vi "Draw Resize Box.vi"(0 "CtrlRef":refnum<vi>, 1 "Corners":refnum<vi>[](array[refnum]), 2 "ID":string, 3 "This VI":refnum<vi>, 5 "Origin":T3, 7 "Coords":T3, 9 "Size":T2, 13 "Active?":bool, 14 "Window Bounds":T1) -> ()   [LabVIEW 2011]
uses:
  <vilib>/Utility/miscctls.llb/LVPoint32TypeDef.ctl
  <vilib>/Utility/miscctls.llb/LVBoundsTypeDef.ctl
  <vilib>/Utility/miscctls.llb/LVRectTypeDef.ctl
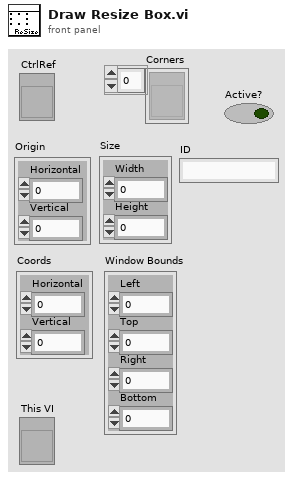
[diagram p1: front panel]
types:
  T1 = typedef "LVRectTypeDef.ctl" = cluster{"Left":i16, "Top":i16, "Right":i16, "Bottom":i16}
  T2 = typedef "LVBoundsTypeDef.ctl" = cluster{"Width":u32, "Height":u32}
  T3 = typedef "LVPoint32TypeDef.ctl" = cluster{"Horizontal":i32, "Vertical":i32}
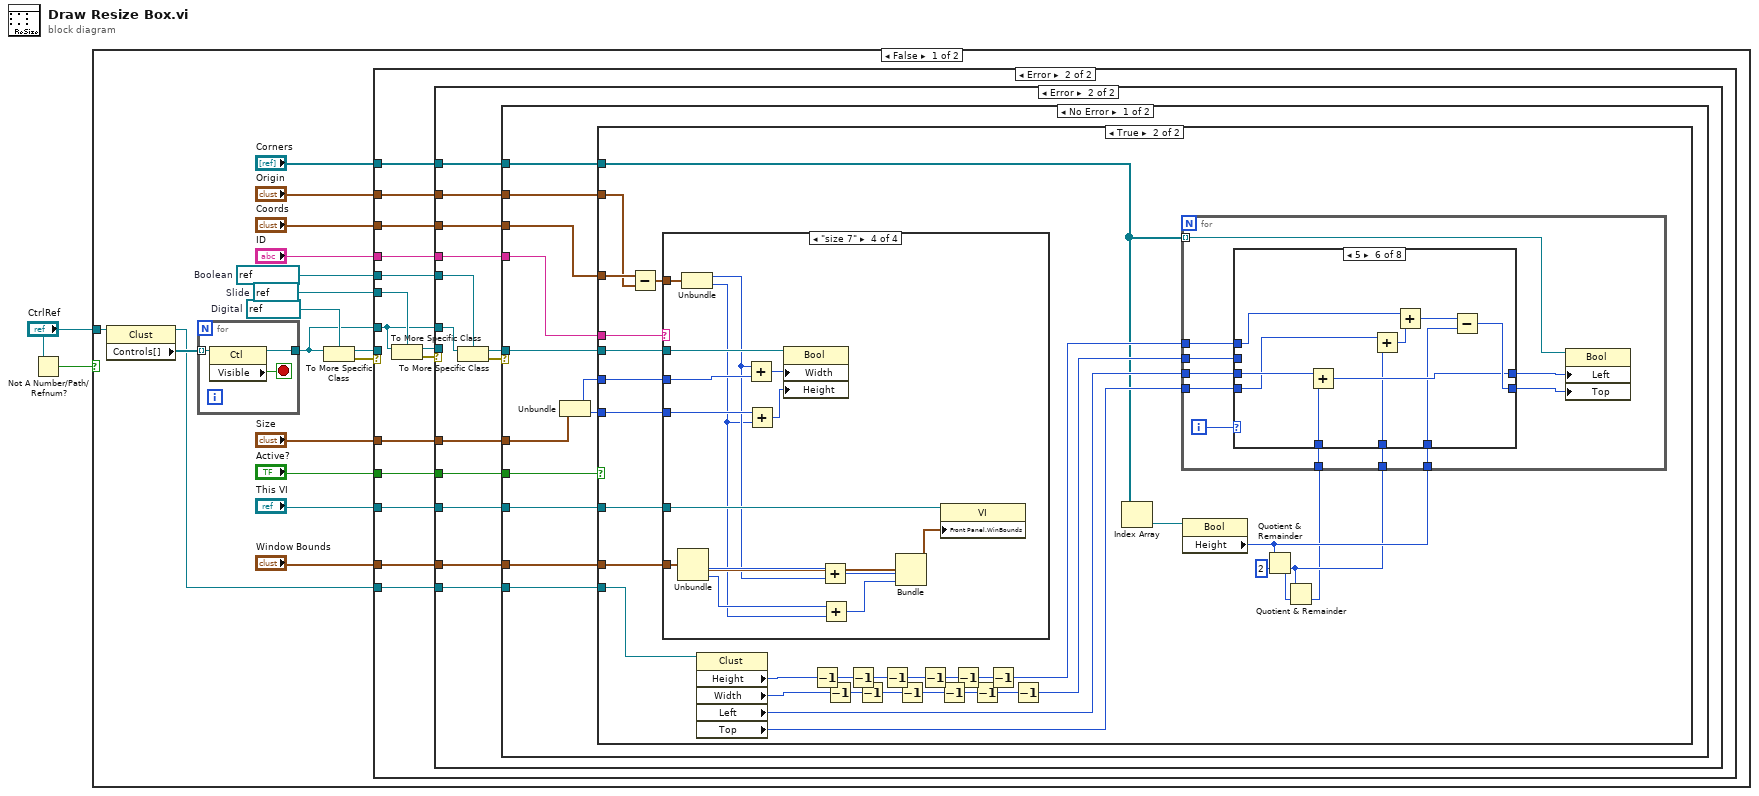
[diagram p0: block diagram]
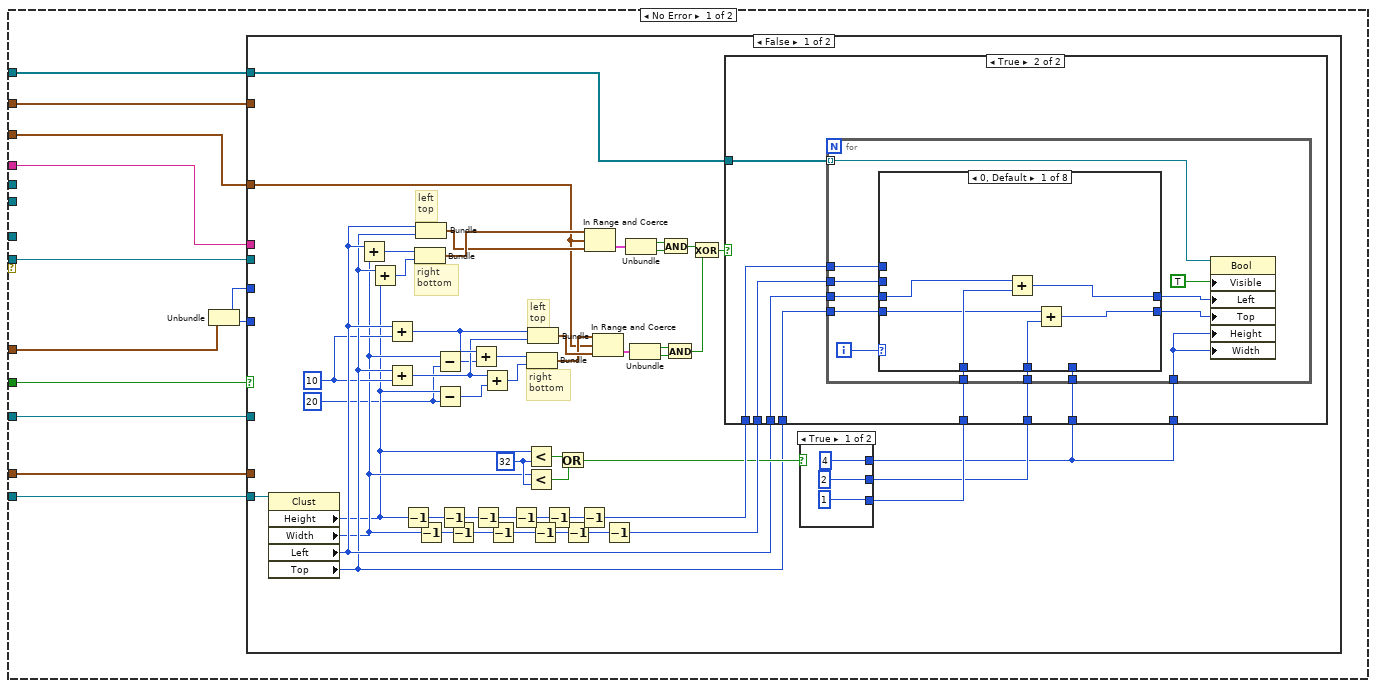
[diagram p2: hidden frame]
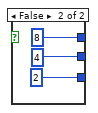
[diagram p3: hidden frame]
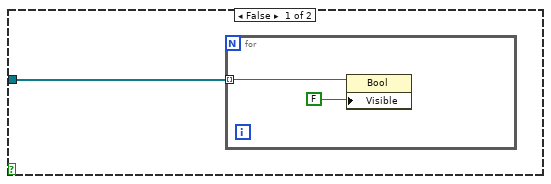
[diagram p4: hidden frame]
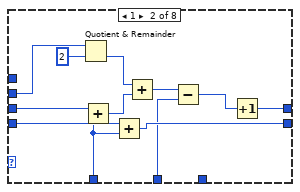
[diagram p5: hidden frame]
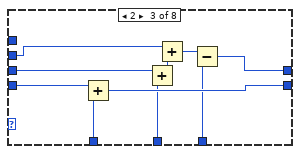
[diagram p6: hidden frame]
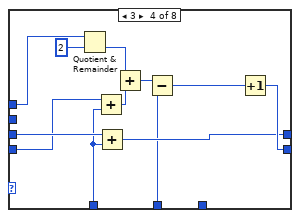
[diagram p7: hidden frame]
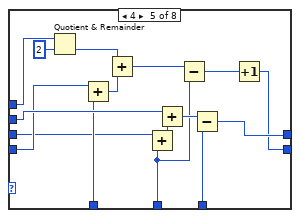
[diagram p8: hidden frame]
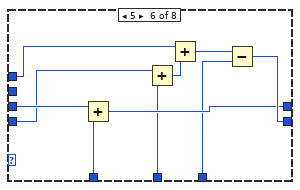
[diagram p9: hidden frame]
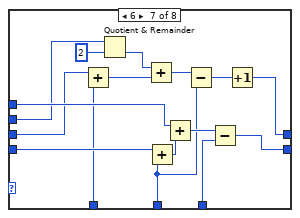
[diagram p10: hidden frame]
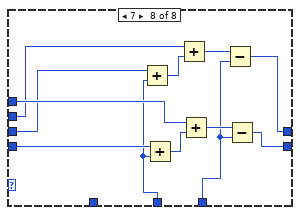
[diagram p11: hidden frame]
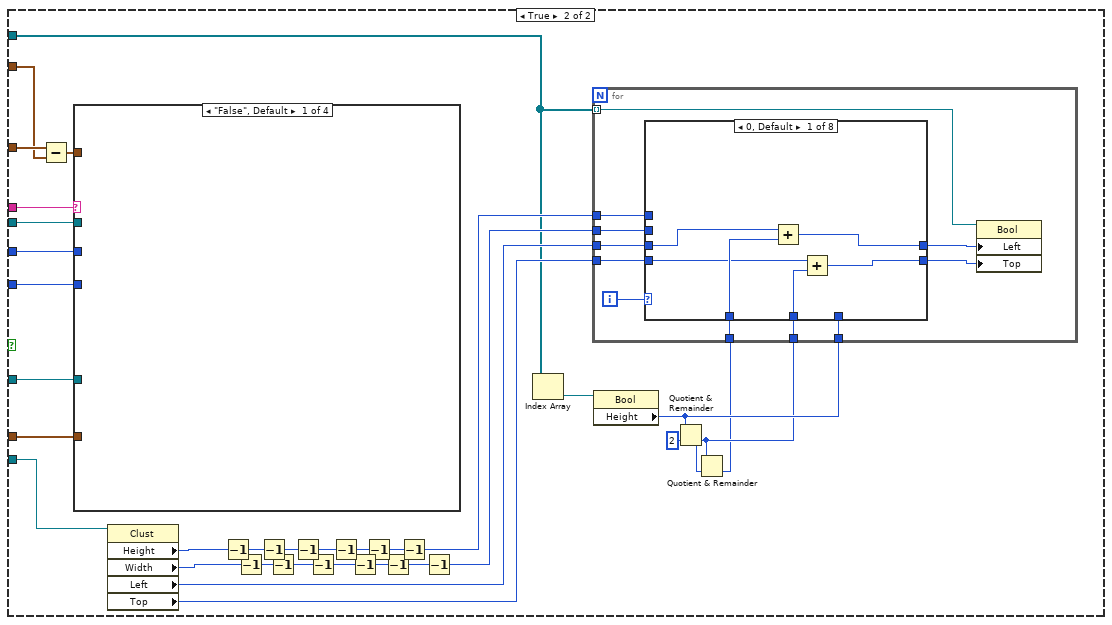
[diagram p12: hidden frame]
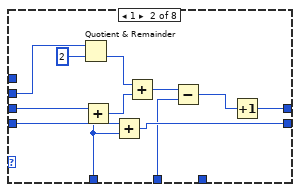
[diagram p13: hidden frame]
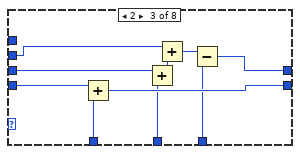
[diagram p14: hidden frame]
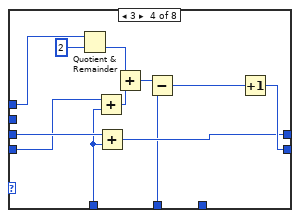
[diagram p15: hidden frame]
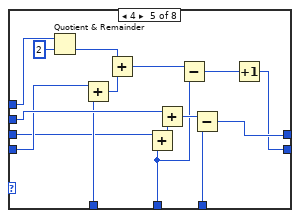
[diagram p16: hidden frame]
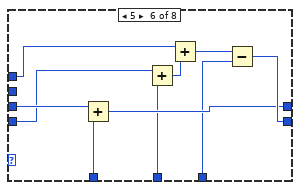
[diagram p17: hidden frame]
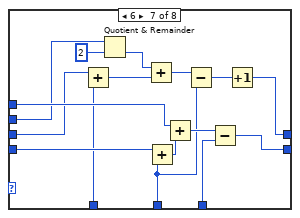
[diagram p18: hidden frame]
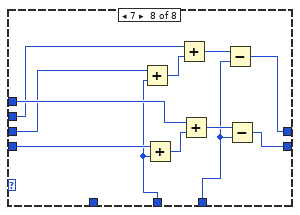
[diagram p19: hidden frame]
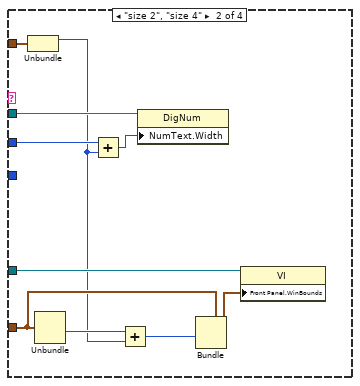
[diagram p20: hidden frame]
diagram:
  n1 = Not A Number/Path/Refnum?(number/path/refnum="CtrlRef") -> (NaN/Path/Refnum?=w1:bool)
  n2 = case shown="False" w1 {
    tunnel: "CtrlRef" -> [w18 _]
    frame False {
      w16 = refnum<vi> refnum  # Boolean
      w15 = refnum<vi> refnum  # Slide
      w14 = refnum<vi> refnum  # Digital
      n3 = property class="Clust"(reference=w18) -> (reference out=w17:refnum<vi>, "Controls[]"=w19:refnum<vi>[])  [unwired: 1 in, 1 out]
      n4 = for {
        tunnel: w19 -> [w1155] mode=indexing
        tunnel: [w1153] -> w13
        stop <- w1154 stop-if-true
        n5 = property class="Ctl"(reference=w1155) -> (reference out=w1153:refnum<vi>, "Visible"=w1154:bool)  [unwired: 1 in, 1 out]
      }
      n6 = To More Specific Class(target class=w14, reference=w13) -> (specific class reference=w11:refnum<vi>, error out=w12:errorcluster)  [unwired: 1 in]
      n7 = case shown="Error" w12 {
        tunnel: w17 -> [w22 w393]
        tunnel: w16 -> [_ w392]
        tunnel: w15 -> [_ w390]
        tunnel: w13 -> [_ w388]
        tunnel: w11 -> [w27 _]
        tunnel: "Corners" -> [w31 w387]
        tunnel: "Origin" -> [w30 w386]
        tunnel: "Coords" -> [w29 w385]
        tunnel: "ID" -> [w28 w384]
        tunnel: "Size" -> [w26 w383]
        tunnel: "Active?" -> [w25 w382]
        tunnel: "This VI" -> [w24 w381]
        tunnel: "Window Bounds" -> [w23 w380]
        frame No Error {
          n8 = Unbundle(w26) -> ("Width"=w21:u32, "Height"=w20:u32)
          n9 = case shown="False" w25 {
            tunnel: w29 -> [w45 w237]
            tunnel: w27 -> [_ w236]
            tunnel: w31 -> [w80 w212]
            tunnel: w28 -> [_ w234]
            tunnel: w21 -> [_ w233]
            tunnel: w20 -> [_ w232]
            tunnel: w24 -> [_ w231]
            tunnel: w23 -> [_ w230]
            tunnel: w22 -> [w74 w217]
            tunnel: w30 -> [_ w206]
            frame False {
              w35 = u32 20 ("y")
              w40 = u32 10 ("y")
              w59 = u32 32 ("y")
              # "right\nbottom"
              # "left\ntop"
              # "right\nbottom"
              # "left\ntop"
              n10 = property class="Clust"(reference=w74) -> ("Height"=w36:u32, "Width"=w37:u32, "Left"=w44:i32, "Top"=w42:i32)  [unwired: 1 in, 2 out]
              n11 = Add(x=w44, y=w37) -> (x+y=w61:u32)
              n12 = Add(x=w42, y=w36) -> (x+y=w60:u32)
              n13 = Add(x=w44, y=w40) -> (x+y=w43:u32)
              n14 = Add(x=w42, y=w40) -> (x+y=w41:u32)
              n15 = Decrement(x=w36) -> (x-1=w73:u32)
              n16 = Bundle(w61, w60) -> (w79:cluster{u32, u32})  [unwired: 1 in]
              n17 = Bundle("Left"=w44, "Top"=w42) -> (w78:cluster{"Left":i32, "Top":i32})  [unwired: 1 in]
              n18 = Decrement(x=w37) -> (x-1=w69:u32)
              n19 = Subtract(x=w37, y=w35) -> (x-y=w39:u32)
              n20 = Subtract(x=w36, y=w35) -> (x-y=w38:u32)
              n21 = Decrement(x=w73) -> (x-1=w72:u32)
              n22 = Decrement(x=w69) -> (x-1=w68:u32)
              n23 = Add(x=w43, y=w39) -> (x+y=w51:u32)
              n24 = Decrement(x=w72) -> (x-1=w71:u32)
              n25 = Add(x=w41, y=w38) -> (x+y=w52:u32)
              n26 = Decrement(x=w68) -> (x-1=w67:u32)
              n27 = Decrement(x=w71) -> (x-1=w70:u32)
              n28 = Less?(x=w36, y=w59) -> (x < y?=w58:bool)
              n29 = Less?(x=w37, y=w59) -> (x < y?=w57:bool)
              n30 = Bundle(w51, w52) -> (w46:cluster{u32, u32})  [unwired: 1 in]
              n31 = Bundle(w43, w41) -> (w47:cluster{u32, u32})  [unwired: 1 in]
              n32 = Decrement(x=w67) -> (x-1=w66:u32)
              n33 = Decrement(x=w70) -> (x-1=w65:u32)
              n34 = Or(x=w58, y=w57) -> (x .or. y?=w56:bool)
              n35 = Decrement(x=w66) -> (x-1=w63:u32)
              n36 = Decrement(x=w65) -> (x-1=w64:u32)
              n37 = In Range and Coerce(upper limit=w79, x=w45, lower limit=w78) -> (In Range?=w77:cluster{"Horizontal":bool, "Vertical":bool})  [unwired: 1 out]
              n38 = In Range and Coerce(upper limit=w46, x=w45, lower limit=w47) -> (In Range?=w48:cluster{"Horizontal":bool, "Vertical":bool})  [unwired: 1 out]
              n39 = Decrement(x=w63) -> (x-1=w62:u32)
              n40 = Unbundle(w77) -> ("Horizontal"=w76:bool, "Vertical"=w75:bool)
              n41 = Unbundle(w48) -> ("Horizontal"=w49:bool, "Vertical"=w50:bool)
              n42 = And(x=w76, y=w75) -> (x .and. y?=w33:bool)
              n43 = And(x=w49, y=w50) -> (x .and. y?=w32:bool)
              n44 = Exclusive Or(1:w32, 2:w33) -> (0:w34:bool)
              n45 = case shown="True" w56 {
                tunnel: [u32 1 ("y") u32 2 ("y")] -> w55
                tunnel: [u32 4 ("y") u32 8 ("y")] -> w53
                tunnel: [u32 2 ("y") u32 4 ("y")] -> w54
                frame True {
                }
                frame False {
                }
              }
              n46 = case shown="True" w34 {
                tunnel: w80 -> [w87 w98]
                tunnel: w64 -> [_ w97]
                tunnel: w62 -> [_ w96]
                tunnel: w44 -> [_ w95]
                tunnel: w42 -> [_ w94]
                tunnel: w55 -> [_ w93]
                tunnel: w53 -> [_ w92]
                tunnel: w54 -> [_ w91]
                tunnel: w53 -> [_ w90]
                frame False {
                  n47 = for {
                    tunnel: w87 -> [w89] mode=indexing
                    n48 = property class="Bool"(reference=w89, "Visible"=FALSE) -> ()  [unwired: 1 in, 2 out]
                  }
                }
                frame True {
                  n49 = for {
                    tunnel: w98 -> [w111] mode=indexing
                    tunnel: w95 -> [w108]
                    tunnel: w94 -> [w106]
                    tunnel: w97 -> [w105]
                    tunnel: w96 -> [w104]
                    tunnel: w93 -> [w102]
                    tunnel: w92 -> [w101]
                    tunnel: w91 -> [w100]
                    tunnel: w90 -> [w99]
                    i -> [w110]
                    n50 = case shown="0, Default" w110 {
                      tunnel: [w117 w124 w136 w142 w166 w172 w186 w201] -> w109
                      tunnel: w108 -> [w113 w123 w131 w144 w155 w174 w179 w199]
                      tunnel: [w116 w120 w139 w147 w160 w175 w191 w203] -> w107
                      tunnel: w106 -> [w112 w122 w134 w143 w157 w171 w183 w197]
                      tunnel: w105 -> [_ _ _ w146 w159 w176 w192 w204]
                      tunnel: w104 -> [_ w127 w137 _ w165 _ w185 w200]
                      tunnel: w102 -> [w115 w119 w133 w141 w156 w173 w178 _]
                      tunnel: w100 -> [w114 w118 w130 w140 w153 w170 w181 w194]
                      tunnel: w99 -> [_ _ w135 _ w152 w168 w182 w196]
                      frame 0, Default {
                        n51 = Add(x=w113, y=w115) -> (x+y=w117:u32)
                        n52 = Add(x=w112, y=w114) -> (x+y=w116:u32)
                      }
                      frame 1 {
                        n53 = Quotient & Remainder(x=w127, y=u32 2) -> (floor(x/y)=w125:u32)  [unwired: 1 out]
                        n54 = Add(x=w123, y=w119) -> (x+y=w121:u32)
                        n55 = Add(x=w122, y=w119) -> (x+y=w120:u32)
                        n56 = Add(x=w125, y=w121) -> (x+y=w129:u32)
                        n57 = Subtract(x=w129, y=w118) -> (x-y=w128:u32)
                        n58 = Increment(x=w128) -> (x+1=w124:u32)
                      }
                      frame 2 {
                        n59 = Add(x=w134, y=w133) -> (x+y=w139:u32)
                        n60 = Add(x=w131, y=w130) -> (x+y=w132:u32)
                        n61 = Add(x=w137, y=w132) -> (x+y=w138:u32)
                        n62 = Subtract(x=w138, y=w135) -> (x-y=w136:u32)
                      }
                      frame 3 {
                        n63 = Quotient & Remainder(x=w146, y=u32 2) -> (floor(x/y)=w148:u32)  [unwired: 1 out]
                        n64 = Add(x=w143, y=w141) -> (x+y=w145:u32)
                        n65 = Add(x=w144, y=w141) -> (x+y=w142:u32)
                        n66 = Add(x=w148, y=w145) -> (x+y=w151:u32)
                        n67 = Subtract(x=w151, y=w140) -> (x-y=w150:u32)
                        n68 = Increment(x=w150) -> (x+1=w147:u32)
                      }
                      frame 4 {
                        n69 = Quotient & Remainder(x=w159, y=u32 2) -> (floor(x/y)=w161:u32)  [unwired: 1 out]
                        n70 = Add(x=w157, y=w156) -> (x+y=w158:u32)
                        n71 = Add(x=w161, y=w158) -> (x+y=w164:u32)
                        n72 = Add(x=w155, y=w153) -> (x+y=w154:u32)
                        n73 = Add(x=w165, y=w154) -> (x+y=w167:u32)
                        n74 = Subtract(x=w164, y=w153) -> (x-y=w163:u32)
                        n75 = Subtract(x=w167, y=w152) -> (x-y=w166:u32)
                        n76 = Increment(x=w163) -> (x+1=w160:u32)
                      }
                      frame 5 {
                        n77 = Add(x=w174, y=w173) -> (x+y=w172:u32)
                        n78 = Add(x=w171, y=w170) -> (x+y=w169:u32)
                        n79 = Add(x=w176, y=w169) -> (x+y=w177:u32)
                        n80 = Subtract(x=w177, y=w168) -> (x-y=w175:u32)
                      }
                      frame 6 {
                        n81 = Add(x=w179, y=w178) -> (x+y=w180:u32)
                        n82 = Quotient & Remainder(x=w185, y=u32 2) -> (floor(x/y)=w187:u32)  [unwired: 1 out]
                        n83 = Add(x=w187, y=w180) -> (x+y=w190:u32)
                        n84 = Add(x=w183, y=w181) -> (x+y=w184:u32)
                        n85 = Add(x=w192, y=w184) -> (x+y=w193:u32)
                        n86 = Subtract(x=w190, y=w181) -> (x-y=w189:u32)
                        n87 = Subtract(x=w193, y=w182) -> (x-y=w191:u32)
                        n88 = Increment(x=w189) -> (x+1=w186:u32)
                      }
                      frame 7 {
                        n89 = Add(x=w199, y=w194) -> (x+y=w198:u32)
                        n90 = Add(x=w197, y=w194) -> (x+y=w195:u32)
                        n91 = Add(x=w200, y=w198) -> (x+y=w202:u32)
                        n92 = Add(x=w204, y=w195) -> (x+y=w205:u32)
                        n93 = Subtract(x=w202, y=w196) -> (x-y=w201:u32)
                        n94 = Subtract(x=w205, y=w196) -> (x-y=w203:u32)
                      }
                    }
                    n95 = property class="Bool"(reference=w111, "Visible"=TRUE, "Left"=w109, "Top"=w107, "Height"=w101, "Width"=w101) -> ()  [unwired: 1 in, 2 out]
                  }
                }
              }
            }
            frame True {
              w209 = u32 2 ("y")
              n96 = Subtract(x=w237, y=w206) -> (x-y=w235:T3)
              n97 = case shown="\"False\", Default" w234 {
                tunnel: w236 -> [_ w350 w356 w378]
                tunnel: w235 -> [_ w352 w363 w379]
                tunnel: w233 -> [_ w349 _ w375]
                tunnel: w232 -> [_ _ w362 w377]
                tunnel: w231 -> [_ w348 w360 w372]
                tunnel: w230 -> [_ w347 w359 w371]
                frame "False", Default {
                }
                frame "size 2", "size 4" {
                  n98 = Unbundle(w352) -> ("Horizontal"=w344:i32)  [unwired: 1 out]
                  n99 = Unbundle(w347) -> ("Right"=w345:i16)  [unwired: 3 out]
                  n100 = Add(x=w349, y=w344) -> (x+y=w351:u32)
                  n101 = Add(x=w345, y=w344) -> (x+y=w343:i32)
                  n102 = property class="DigNum"(reference=w350, "NumText.Width"=w351) -> ()  [unwired: 1 in, 2 out]
                  n103 = Bundle(cluster=w347, "Right"=w343) -> (w346:T1)  [unwired: 3 in]
                  n104 = property class="VI"(reference=w348, "Front Panel.WinBounds"=w346) -> ()  [unwired: 1 in, 2 out]
                }
                frame "size 6" {
                  n105 = Unbundle(w363) -> ("Vertical"=w358:i32)  [unwired: 1 out]
                  n106 = Unbundle(w359) -> ("Bottom"=w357:i16)  [unwired: 3 out]
                  n107 = Add(x=w362, y=w358) -> (x+y=w354:u32)
                  n108 = call "Get Font Size.vi"("Height"=w354) -> ("Font Size"=w353:i32)  [unwired: 14 in]
                  n109 = Add(x=w357, y=w358) -> (x+y=w355:i32)
                  n110 = property class="DigNum"(reference=w356, "NumText.Height"=w354, "NumText.FontSize"=w353) -> ()  [unwired: 1 in, 2 out]
                  n111 = Bundle(cluster=w359, "Bottom"=w355) -> (w361:T1)  [unwired: 3 in]
                  n112 = property class="VI"(reference=w360, "Front Panel.WinBounds"=w361) -> ()  [unwired: 1 in, 2 out]
                }
                frame "size 7" {
                  n113 = Unbundle(w371) -> ("Right"=w373:i16, "Bottom"=w369:i16)  [unwired: 2 out]
                  n114 = Unbundle(w379) -> ("Horizontal"=w368:i32, "Vertical"=w367:i32)
                  n115 = Add(x=w368, y=w375) -> (x+y=w376:u32)
                  n116 = Add(x=w377, y=w367) -> (x+y=w365:u32)
                  n117 = Add(x=w373, y=w368) -> (x+y=w370:i32)
                  n118 = Add(x=w369, y=w367) -> (x+y=w366:i32)
                  n119 = call "Get Font Size.vi"("Height"=w365) -> ("Font Size"=w364:i32)  [unwired: 14 in]
                  n120 = Bundle(cluster=w371, "Right"=w370, "Bottom"=w366) -> (w374:T1)  [unwired: 2 in]
                  n121 = property class="DigNum"(reference=w378, "NumText.Width"=w376, "NumText.Height"=w365, "NumText.FontSize"=w364) -> ()  [unwired: 1 in, 2 out]
                  n122 = property class="VI"(reference=w372, "Front Panel.WinBounds"=w374) -> ()  [unwired: 1 in, 2 out]
                }
              }
              n123 = property class="Clust"(reference=w217) -> ("Height"=w229:u32, "Width"=w228:u32, "Left"=w214:i32, "Top"=w213:i32)  [unwired: 1 in, 2 out]
              n124 = Decrement(x=w229) -> (x-1=w227:u32)
              n125 = Decrement(x=w228) -> (x-1=w223:u32)
              n126 = Decrement(x=w227) -> (x-1=w226:u32)
              n127 = Decrement(x=w223) -> (x-1=w222:u32)
              n128 = Decrement(x=w226) -> (x-1=w225:u32)
              n129 = Decrement(x=w222) -> (x-1=w221:u32)
              n130 = Decrement(x=w225) -> (x-1=w224:u32)
              n131 = Decrement(x=w221) -> (x-1=w220:u32)
              n132 = Decrement(x=w224) -> (x-1=w219:u32)
              n133 = Decrement(x=w220) -> (x-1=w218:u32)
              n134 = Decrement(x=w219) -> (x-1=w216:u32)
              n135 = Decrement(x=w218) -> (x-1=w215:u32)
              n136 = Index Array(array=w212) -> (element=w211:refnum<vi>)  [unwired: 1 in]
              n137 = property class="Bool"(reference=w211) -> ("Height"=w210:u32)  [unwired: 1 in, 2 out]
              n138 = Quotient & Remainder(x=w210, y=w209) -> (floor(x/y)=w208:u32)  [unwired: 1 out]
              n139 = Quotient & Remainder(x=w208, y=w209) -> (floor(x/y)=w207:u32)  [unwired: 1 out]
              n140 = for {
                tunnel: w212 -> [w248] mode=indexing
                tunnel: w214 -> [w245]
                tunnel: w213 -> [w243]
                tunnel: w216 -> [w242]
                tunnel: w215 -> [w241]
                tunnel: w207 -> [w240]
                tunnel: w208 -> [w239]
                tunnel: w210 -> [w238]
                i -> [w247]
                n141 = case shown="0, Default" w247 {
                  tunnel: [w254 w261 w273 w279 w303 w309 w323 w338] -> w246
                  tunnel: w245 -> [w250 w260 w268 w281 w292 w311 w316 w336]
                  tunnel: [w253 w257 w276 w284 w297 w312 w328 w340] -> w244
                  tunnel: w243 -> [w249 w259 w271 w280 w294 w308 w320 w334]
                  tunnel: w242 -> [_ _ _ w283 w296 w313 w329 w341]
                  tunnel: w241 -> [_ w264 w274 _ w302 _ w322 w337]
                  tunnel: w240 -> [w252 w256 w270 w278 w293 w310 w315 _]
                  tunnel: w239 -> [w251 w255 w267 w277 w290 w307 w318 w331]
                  tunnel: w238 -> [_ _ w272 _ w289 w305 w319 w333]
                  frame 0, Default {
                    n142 = Add(x=w250, y=w252) -> (x+y=w254:u32)
                    n143 = Add(x=w249, y=w251) -> (x+y=w253:u32)
                  }
                  frame 1 {
                    n144 = Quotient & Remainder(x=w264, y=u32 2) -> (floor(x/y)=w262:u32)  [unwired: 1 out]
                    n145 = Add(x=w260, y=w256) -> (x+y=w258:u32)
                    n146 = Add(x=w259, y=w256) -> (x+y=w257:u32)
                    n147 = Add(x=w262, y=w258) -> (x+y=w266:u32)
                    n148 = Subtract(x=w266, y=w255) -> (x-y=w265:u32)
                    n149 = Increment(x=w265) -> (x+1=w261:u32)
                  }
                  frame 2 {
                    n150 = Add(x=w271, y=w270) -> (x+y=w276:u32)
                    n151 = Add(x=w268, y=w267) -> (x+y=w269:u32)
                    n152 = Add(x=w274, y=w269) -> (x+y=w275:u32)
                    n153 = Subtract(x=w275, y=w272) -> (x-y=w273:u32)
                  }
                  frame 3 {
                    n154 = Quotient & Remainder(x=w283, y=u32 2) -> (floor(x/y)=w285:u32)  [unwired: 1 out]
                    n155 = Add(x=w280, y=w278) -> (x+y=w282:u32)
                    n156 = Add(x=w281, y=w278) -> (x+y=w279:u32)
                    n157 = Add(x=w285, y=w282) -> (x+y=w288:u32)
                    n158 = Subtract(x=w288, y=w277) -> (x-y=w287:u32)
                    n159 = Increment(x=w287) -> (x+1=w284:u32)
                  }
                  frame 4 {
                    n160 = Quotient & Remainder(x=w296, y=u32 2) -> (floor(x/y)=w298:u32)  [unwired: 1 out]
                    n161 = Add(x=w294, y=w293) -> (x+y=w295:u32)
                    n162 = Add(x=w298, y=w295) -> (x+y=w301:u32)
                    n163 = Add(x=w292, y=w290) -> (x+y=w291:u32)
                    n164 = Add(x=w302, y=w291) -> (x+y=w304:u32)
                    n165 = Subtract(x=w301, y=w290) -> (x-y=w300:u32)
                    n166 = Subtract(x=w304, y=w289) -> (x-y=w303:u32)
                    n167 = Increment(x=w300) -> (x+1=w297:u32)
                  }
                  frame 5 {
                    n168 = Add(x=w311, y=w310) -> (x+y=w309:u32)
                    n169 = Add(x=w308, y=w307) -> (x+y=w306:u32)
                    n170 = Add(x=w313, y=w306) -> (x+y=w314:u32)
                    n171 = Subtract(x=w314, y=w305) -> (x-y=w312:u32)
                  }
                  frame 6 {
                    n172 = Add(x=w316, y=w315) -> (x+y=w317:u32)
                    n173 = Quotient & Remainder(x=w322, y=u32 2) -> (floor(x/y)=w324:u32)  [unwired: 1 out]
                    n174 = Add(x=w324, y=w317) -> (x+y=w327:u32)
                    n175 = Add(x=w320, y=w318) -> (x+y=w321:u32)
                    n176 = Add(x=w329, y=w321) -> (x+y=w330:u32)
                    n177 = Subtract(x=w327, y=w318) -> (x-y=w326:u32)
                    n178 = Subtract(x=w330, y=w319) -> (x-y=w328:u32)
                    n179 = Increment(x=w326) -> (x+1=w323:u32)
                  }
                  frame 7 {
                    n180 = Add(x=w336, y=w331) -> (x+y=w335:u32)
                    n181 = Add(x=w334, y=w331) -> (x+y=w332:u32)
                    n182 = Add(x=w337, y=w335) -> (x+y=w339:u32)
                    n183 = Add(x=w341, y=w332) -> (x+y=w342:u32)
                    n184 = Subtract(x=w339, y=w333) -> (x-y=w338:u32)
                    n185 = Subtract(x=w342, y=w333) -> (x-y=w340:u32)
                  }
                }
                n186 = property class="Bool"(reference=w248, "Left"=w246, "Top"=w244) -> ()  [unwired: 1 in, 2 out]
              }
            }
          }
        }
        frame Error {
          n187 = To More Specific Class(target class=w390, reference=w388) -> (specific class reference=w389:refnum<vi>, error out=w391:errorcluster)  [unwired: 1 in]
          n188 = case shown="Error" w391 {
            tunnel: w388 -> [_ w793]
            tunnel: w393 -> [w395 w792]
            tunnel: w392 -> [_ w791]
            tunnel: w389 -> [w394 _]
            tunnel: w387 -> [w403 w790]
            tunnel: w386 -> [w402 w789]
            tunnel: w385 -> [w401 w788]
            tunnel: w384 -> [w400 w787]
            tunnel: w383 -> [w399 w786]
            tunnel: w382 -> [w398 w785]
            tunnel: w381 -> [w397 w784]
            tunnel: w380 -> [w396 w783]
            frame No Error {
              n189 = Unbundle(w399) -> ("Width"=w405:u32, "Height"=w404:u32)
              n190 = case shown="True" w398 {
                tunnel: w401 -> [w419 w611]
                tunnel: w394 -> [_ w610]
                tunnel: w403 -> [w454 w586]
                tunnel: w400 -> [_ w608]
                tunnel: w405 -> [_ w607]
                tunnel: w404 -> [_ w606]
                tunnel: w397 -> [_ w605]
                tunnel: w396 -> [_ w604]
                tunnel: w395 -> [w448 w591]
                tunnel: w402 -> [_ w580]
                frame False {
                  w409 = u32 20 ("y")
                  w414 = u32 10 ("y")
                  w433 = u32 32 ("y")
                  # "right\nbottom"
                  # "left\ntop"
                  # "right\nbottom"
                  # "left\ntop"
                  n191 = property class="Clust"(reference=w448) -> ("Height"=w410:u32, "Width"=w411:u32, "Left"=w418:i32, "Top"=w416:i32)  [unwired: 1 in, 2 out]
                  n192 = Add(x=w418, y=w411) -> (x+y=w435:u32)
                  n193 = Add(x=w416, y=w410) -> (x+y=w434:u32)
                  n194 = Add(x=w418, y=w414) -> (x+y=w417:u32)
                  n195 = Add(x=w416, y=w414) -> (x+y=w415:u32)
                  n196 = Decrement(x=w410) -> (x-1=w447:u32)
                  n197 = Bundle(w435, w434) -> (w453:cluster{u32, u32})  [unwired: 1 in]
                  n198 = Bundle("Left"=w418, "Top"=w416) -> (w452:cluster{"Left":i32, "Top":i32})  [unwired: 1 in]
                  n199 = Decrement(x=w411) -> (x-1=w443:u32)
                  n200 = Subtract(x=w411, y=w409) -> (x-y=w413:u32)
                  n201 = Subtract(x=w410, y=w409) -> (x-y=w412:u32)
                  n202 = Decrement(x=w447) -> (x-1=w446:u32)
                  n203 = Decrement(x=w443) -> (x-1=w442:u32)
                  n204 = Add(x=w417, y=w413) -> (x+y=w425:u32)
                  n205 = Decrement(x=w446) -> (x-1=w445:u32)
                  n206 = Add(x=w415, y=w412) -> (x+y=w426:u32)
                  n207 = Decrement(x=w442) -> (x-1=w441:u32)
                  n208 = Decrement(x=w445) -> (x-1=w444:u32)
                  n209 = Less?(x=w410, y=w433) -> (x < y?=w432:bool)
                  n210 = Less?(x=w411, y=w433) -> (x < y?=w431:bool)
                  n211 = Bundle(w425, w426) -> (w420:cluster{u32, u32})  [unwired: 1 in]
                  n212 = Bundle(w417, w415) -> (w421:cluster{u32, u32})  [unwired: 1 in]
                  n213 = Decrement(x=w441) -> (x-1=w440:u32)
                  n214 = Decrement(x=w444) -> (x-1=w439:u32)
                  n215 = Or(x=w432, y=w431) -> (x .or. y?=w430:bool)
                  n216 = Decrement(x=w440) -> (x-1=w437:u32)
                  n217 = Decrement(x=w439) -> (x-1=w438:u32)
                  n218 = In Range and Coerce(upper limit=w453, x=w419, lower limit=w452) -> (In Range?=w451:cluster{"Horizontal":bool, "Vertical":bool})  [unwired: 1 out]
                  n219 = In Range and Coerce(upper limit=w420, x=w419, lower limit=w421) -> (In Range?=w422:cluster{"Horizontal":bool, "Vertical":bool})  [unwired: 1 out]
                  n220 = Decrement(x=w437) -> (x-1=w436:u32)
                  n221 = Unbundle(w451) -> ("Horizontal"=w450:bool, "Vertical"=w449:bool)
                  n222 = Unbundle(w422) -> ("Horizontal"=w423:bool, "Vertical"=w424:bool)
                  n223 = And(x=w450, y=w449) -> (x .and. y?=w407:bool)
                  n224 = And(x=w423, y=w424) -> (x .and. y?=w406:bool)
                  n225 = Exclusive Or(1:w406, 2:w407) -> (0:w408:bool)
                  n226 = case shown="False" w430 {
                    tunnel: [u32 1 ("y") u32 2 ("y")] -> w429
                    tunnel: [u32 4 ("y") u32 8 ("y")] -> w427
                    tunnel: [u32 2 ("y") u32 4 ("y")] -> w428
                    frame True {
                    }
                    frame False {
                    }
                  }
                  n227 = case shown="True" w408 {
                    tunnel: w454 -> [w461 w472]
                    tunnel: w438 -> [_ w471]
                    tunnel: w436 -> [_ w470]
                    tunnel: w418 -> [_ w469]
                    tunnel: w416 -> [_ w468]
                    tunnel: w429 -> [_ w467]
                    tunnel: w427 -> [_ w466]
                    tunnel: w428 -> [_ w465]
                    tunnel: w427 -> [_ w464]
                    frame False {
                      n228 = for {
                        tunnel: w461 -> [w463] mode=indexing
                        n229 = property class="Bool"(reference=w463, "Visible"=FALSE) -> ()  [unwired: 1 in, 2 out]
                      }
                    }
                    frame True {
                      n230 = for {
                        tunnel: w472 -> [w485] mode=indexing
                        tunnel: w469 -> [w482]
                        tunnel: w468 -> [w480]
                        tunnel: w471 -> [w479]
                        tunnel: w470 -> [w478]
                        tunnel: w467 -> [w476]
                        tunnel: w466 -> [w475]
                        tunnel: w465 -> [w474]
                        tunnel: w464 -> [w473]
                        i -> [w484]
                        n231 = case shown="2" w484 {
                          tunnel: [w491 w498 w510 w516 w540 w546 w560 w575] -> w483
                          tunnel: w482 -> [w487 w497 w505 w518 w529 w548 w553 w573]
                          tunnel: [w490 w494 w513 w521 w534 w549 w565 w577] -> w481
                          tunnel: w480 -> [w486 w496 w508 w517 w531 w545 w557 w571]
                          tunnel: w479 -> [_ _ _ w520 w533 w550 w566 w578]
                          tunnel: w478 -> [_ w501 w511 _ w539 _ w559 w574]
                          tunnel: w476 -> [w489 w493 w507 w515 w530 w547 w552 _]
                          tunnel: w474 -> [w488 w492 w504 w514 w527 w544 w555 w568]
                          tunnel: w473 -> [_ _ w509 _ w526 w542 w556 w570]
                          frame 0, Default {
                            n232 = Add(x=w487, y=w489) -> (x+y=w491:u32)
                            n233 = Add(x=w486, y=w488) -> (x+y=w490:u32)
                          }
                          frame 1 {
                            n234 = Quotient & Remainder(x=w501, y=u32 2) -> (floor(x/y)=w499:u32)  [unwired: 1 out]
                            n235 = Add(x=w497, y=w493) -> (x+y=w495:u32)
                            n236 = Add(x=w496, y=w493) -> (x+y=w494:u32)
                            n237 = Add(x=w499, y=w495) -> (x+y=w503:u32)
                            n238 = Subtract(x=w503, y=w492) -> (x-y=w502:u32)
                            n239 = Increment(x=w502) -> (x+1=w498:u32)
                          }
                          frame 2 {
                            n240 = Add(x=w508, y=w507) -> (x+y=w513:u32)
                            n241 = Add(x=w505, y=w504) -> (x+y=w506:u32)
                            n242 = Add(x=w511, y=w506) -> (x+y=w512:u32)
                            n243 = Subtract(x=w512, y=w509) -> (x-y=w510:u32)
                          }
                          frame 3 {
                            n244 = Quotient & Remainder(x=w520, y=u32 2) -> (floor(x/y)=w522:u32)  [unwired: 1 out]
                            n245 = Add(x=w517, y=w515) -> (x+y=w519:u32)
                            n246 = Add(x=w518, y=w515) -> (x+y=w516:u32)
                            n247 = Add(x=w522, y=w519) -> (x+y=w525:u32)
                            n248 = Subtract(x=w525, y=w514) -> (x-y=w524:u32)
                            n249 = Increment(x=w524) -> (x+1=w521:u32)
                          }
                          frame 4 {
                            n250 = Quotient & Remainder(x=w533, y=u32 2) -> (floor(x/y)=w535:u32)  [unwired: 1 out]
                            n251 = Add(x=w531, y=w530) -> (x+y=w532:u32)
                            n252 = Add(x=w535, y=w532) -> (x+y=w538:u32)
                            n253 = Add(x=w529, y=w527) -> (x+y=w528:u32)
                            n254 = Add(x=w539, y=w528) -> (x+y=w541:u32)
                            n255 = Subtract(x=w538, y=w527) -> (x-y=w537:u32)
                            n256 = Subtract(x=w541, y=w526) -> (x-y=w540:u32)
                            n257 = Increment(x=w537) -> (x+1=w534:u32)
                          }
                          frame 5 {
                            n258 = Add(x=w548, y=w547) -> (x+y=w546:u32)
                            n259 = Add(x=w545, y=w544) -> (x+y=w543:u32)
                            n260 = Add(x=w550, y=w543) -> (x+y=w551:u32)
                            n261 = Subtract(x=w551, y=w542) -> (x-y=w549:u32)
                          }
                          frame 6 {
                            n262 = Add(x=w553, y=w552) -> (x+y=w554:u32)
                            n263 = Quotient & Remainder(x=w559, y=u32 2) -> (floor(x/y)=w561:u32)  [unwired: 1 out]
                            n264 = Add(x=w561, y=w554) -> (x+y=w564:u32)
                            n265 = Add(x=w557, y=w555) -> (x+y=w558:u32)
                            n266 = Add(x=w566, y=w558) -> (x+y=w567:u32)
                            n267 = Subtract(x=w564, y=w555) -> (x-y=w563:u32)
                            n268 = Subtract(x=w567, y=w556) -> (x-y=w565:u32)
                            n269 = Increment(x=w563) -> (x+1=w560:u32)
                          }
                          frame 7 {
                            n270 = Add(x=w573, y=w568) -> (x+y=w572:u32)
                            n271 = Add(x=w571, y=w568) -> (x+y=w569:u32)
                            n272 = Add(x=w574, y=w572) -> (x+y=w576:u32)
                            n273 = Add(x=w578, y=w569) -> (x+y=w579:u32)
                            n274 = Subtract(x=w576, y=w570) -> (x-y=w575:u32)
                            n275 = Subtract(x=w579, y=w570) -> (x-y=w577:u32)
                          }
                        }
                        n276 = property class="Bool"(reference=w485, "Visible"=TRUE, "Left"=w483, "Top"=w481, "Height"=w475, "Width"=w475) -> ()  [unwired: 1 in, 2 out]
                      }
                    }
                  }
                }
                frame True {
                  w583 = u32 2 ("y")
                  n277 = Subtract(x=w611, y=w580) -> (x-y=w609:T3)
                  n278 = case shown="\"size 7\"" w608 {
                    tunnel: w610 -> [_ w724 w742 w763]
                    tunnel: w609 -> [_ w725 w743 w764]
                    tunnel: w607 -> [_ w723 _ w761]
                    tunnel: w606 -> [_ _ w741 w762]
                    tunnel: w605 -> [_ w722 w740 w759]
                    tunnel: w604 -> [_ w721 w739 w758]
                    frame "False", Default {
                    }
                    frame "size 2", "size 4" {
                      n279 = Unbundle(w725) -> ("Horizontal"=w719:i32)  [unwired: 1 out]
                      n280 = Unbundle(w721) -> ("Right"=w720:i16)  [unwired: 3 out]
                      n281 = property class="Slide"(reference=w724) -> (reference out=w718:refnum<vi>, "Label.Text"=w717:string)  [unwired: 1 in, 1 out]
                      n282 = case shown="\"HSlide\"" w717 {
                        tunnel: w723 -> [_ w733]
                        tunnel: w722 -> [_ w732]
                        tunnel: w721 -> [_ w731]
                        tunnel: w720 -> [_ w729]
                        tunnel: w719 -> [_ w728]
                        tunnel: w718 -> [_ w726]
                        frame "False", Default {
                        }
                        frame "HSlide" {
                          n283 = Add(x=w733, y=w728) -> (x+y=w734:u32)
                          n284 = Add(x=w729, y=w728) -> (x+y=w727:i32)
                          n285 = Bundle(cluster=w731, "Right"=w727) -> (w730:T1)  [unwired: 3 in]
                          n286 = property class="Slide"(reference=w726, "Width"=w734) -> ()  [unwired: 1 in, 2 out]
                          n287 = property class="VI"(reference=w732, "Front Panel.WinBounds"=w730) -> ()  [unwired: 1 in, 2 out]
                        }
                      }
                    }
                    frame "size 6" {
                      n288 = Unbundle(w743) -> ("Vertical"=w738:i32)  [unwired: 1 out]
                      n289 = Unbundle(w739) -> ("Bottom"=w736:i16)  [unwired: 3 out]
                      n290 = property class="Slide"(reference=w742) -> (reference out=w737:refnum<vi>, "Label.Text"=w735:string)  [unwired: 1 in, 1 out]
                      n291 = case shown="\"VSlide\"" w735 {
                        tunnel: w741 -> [_ w751]
                        tunnel: w740 -> [_ w749]
                        tunnel: w739 -> [_ w748]
                        tunnel: w738 -> [_ w747]
                        tunnel: w737 -> [_ w745]
                        tunnel: w736 -> [_ w744]
                        frame "False", Default {
                        }
                        frame "VSlide" {
                          n292 = Add(x=w751, y=w747) -> (x+y=w752:u32)
                          n293 = Add(x=w744, y=w747) -> (x+y=w746:i32)
                          n294 = property class="Slide"(reference=w745, "Height"=w752) -> ()  [unwired: 1 in, 2 out]
                          n295 = Bundle(cluster=w748, "Bottom"=w746) -> (w750:T1)  [unwired: 3 in]
                          n296 = property class="VI"(reference=w749, "Front Panel.WinBounds"=w750) -> ()  [unwired: 1 in, 2 out]
                        }
                      }
                    }
                    frame "size 7" {
                      n297 = Unbundle(w758) -> ("Right"=w760:i16, "Bottom"=w757:i16)  [unwired: 2 out]
                      n298 = Unbundle(w764) -> ("Horizontal"=w756:i32, "Vertical"=w755:i32)
                      n299 = property class="Slide"(reference=w763) -> (reference out=w754:refnum<vi>, "Label.Text"=w753:string)  [unwired: 1 in, 1 out]
                      n300 = case shown="\"VSlide\"" w753 {
                        tunnel: w762 -> [_ w773 _]
                        tunnel: w761 -> [_ _ w781]
                        tunnel: w760 -> [_ _ w779]
                        tunnel: w759 -> [_ w771 w778]
                        tunnel: w758 -> [_ w770 w777]
                        tunnel: w757 -> [_ w769 _]
                        tunnel: w756 -> [_ _ w775]
                        tunnel: w755 -> [_ w768 _]
                        tunnel: w754 -> [_ w767 w774]
                        frame "False", Default {
                        }
                        frame "VSlide" {
                          n301 = Add(x=w769, y=w768) -> (x+y=w765:i32)
                          n302 = Add(x=w773, y=w768) -> (x+y=w766:u32)
                          n303 = Bundle(cluster=w770, "Bottom"=w765) -> (w772:T1)  [unwired: 3 in]
                          n304 = property class="Slide"(reference=w767, "Height"=w766) -> ()  [unwired: 1 in, 2 out]
                          n305 = property class="VI"(reference=w771, "Front Panel.WinBounds"=w772) -> ()  [unwired: 1 in, 2 out]
                        }
                        frame "HSlide" {
                          n306 = Add(x=w779, y=w775) -> (x+y=w776:i32)
                          n307 = Add(x=w775, y=w781) -> (x+y=w782:u32)
                          n308 = Bundle(cluster=w777, "Right"=w776) -> (w780:T1)  [unwired: 3 in]
                          n309 = property class="Slide"(reference=w774, "Width"=w782) -> ()  [unwired: 1 in, 2 out]
                          n310 = property class="VI"(reference=w778, "Front Panel.WinBounds"=w780) -> ()  [unwired: 1 in, 2 out]
                        }
                      }
                    }
                  }
                  n311 = property class="Clust"(reference=w591) -> ("Height"=w603:u32, "Width"=w602:u32, "Left"=w588:i32, "Top"=w587:i32)  [unwired: 1 in, 2 out]
                  n312 = Decrement(x=w603) -> (x-1=w601:u32)
                  n313 = Decrement(x=w602) -> (x-1=w597:u32)
                  n314 = Decrement(x=w601) -> (x-1=w600:u32)
                  n315 = Decrement(x=w597) -> (x-1=w596:u32)
                  n316 = Decrement(x=w600) -> (x-1=w599:u32)
                  n317 = Decrement(x=w596) -> (x-1=w595:u32)
                  n318 = Decrement(x=w599) -> (x-1=w598:u32)
                  n319 = Decrement(x=w595) -> (x-1=w594:u32)
                  n320 = Decrement(x=w598) -> (x-1=w593:u32)
                  n321 = Decrement(x=w594) -> (x-1=w592:u32)
                  n322 = Decrement(x=w593) -> (x-1=w590:u32)
                  n323 = Decrement(x=w592) -> (x-1=w589:u32)
                  n324 = Index Array(array=w586) -> (element=w585:refnum<vi>)  [unwired: 1 in]
                  n325 = property class="Bool"(reference=w585) -> ("Height"=w584:u32)  [unwired: 1 in, 2 out]
                  n326 = Quotient & Remainder(x=w584, y=w583) -> (floor(x/y)=w582:u32)  [unwired: 1 out]
                  n327 = Quotient & Remainder(x=w582, y=w583) -> (floor(x/y)=w581:u32)  [unwired: 1 out]
                  n328 = for {
                    tunnel: w586 -> [w622] mode=indexing
                    tunnel: w588 -> [w619]
                    tunnel: w587 -> [w617]
                    tunnel: w590 -> [w616]
                    tunnel: w589 -> [w615]
                    tunnel: w581 -> [w614]
                    tunnel: w582 -> [w613]
                    tunnel: w584 -> [w612]
                    i -> [w621]
                    n329 = case shown="0, Default" w621 {
                      tunnel: [w628 w635 w647 w653 w677 w683 w697 w712] -> w620
                      tunnel: w619 -> [w624 w634 w642 w655 w666 w685 w690 w710]
                      tunnel: [w627 w631 w650 w658 w671 w686 w702 w714] -> w618
                      tunnel: w617 -> [w623 w633 w645 w654 w668 w682 w694 w708]
                      tunnel: w616 -> [_ _ _ w657 w670 w687 w703 w715]
                      tunnel: w615 -> [_ w638 w648 _ w676 _ w696 w711]
                      tunnel: w614 -> [w626 w630 w644 w652 w667 w684 w689 _]
                      tunnel: w613 -> [w625 w629 w641 w651 w664 w681 w692 w705]
                      tunnel: w612 -> [_ _ w646 _ w663 w679 w693 w707]
                      frame 0, Default {
                        n330 = Add(x=w624, y=w626) -> (x+y=w628:u32)
                        n331 = Add(x=w623, y=w625) -> (x+y=w627:u32)
                      }
                      frame 1 {
                        n332 = Quotient & Remainder(x=w638, y=u32 2) -> (floor(x/y)=w636:u32)  [unwired: 1 out]
                        n333 = Add(x=w634, y=w630) -> (x+y=w632:u32)
                        n334 = Add(x=w633, y=w630) -> (x+y=w631:u32)
                        n335 = Add(x=w636, y=w632) -> (x+y=w640:u32)
                        n336 = Subtract(x=w640, y=w629) -> (x-y=w639:u32)
                        n337 = Increment(x=w639) -> (x+1=w635:u32)
                      }
                      frame 2 {
                        n338 = Add(x=w645, y=w644) -> (x+y=w650:u32)
                        n339 = Add(x=w642, y=w641) -> (x+y=w643:u32)
                        n340 = Add(x=w648, y=w643) -> (x+y=w649:u32)
                        n341 = Subtract(x=w649, y=w646) -> (x-y=w647:u32)
                      }
                      frame 3 {
                        n342 = Quotient & Remainder(x=w657, y=u32 2) -> (floor(x/y)=w659:u32)  [unwired: 1 out]
                        n343 = Add(x=w654, y=w652) -> (x+y=w656:u32)
                        n344 = Add(x=w655, y=w652) -> (x+y=w653:u32)
                        n345 = Add(x=w659, y=w656) -> (x+y=w662:u32)
                        n346 = Subtract(x=w662, y=w651) -> (x-y=w661:u32)
                        n347 = Increment(x=w661) -> (x+1=w658:u32)
                      }
                      frame 4 {
                        n348 = Quotient & Remainder(x=w670, y=u32 2) -> (floor(x/y)=w672:u32)  [unwired: 1 out]
                        n349 = Add(x=w668, y=w667) -> (x+y=w669:u32)
                        n350 = Add(x=w672, y=w669) -> (x+y=w675:u32)
                        n351 = Add(x=w666, y=w664) -> (x+y=w665:u32)
                        n352 = Add(x=w676, y=w665) -> (x+y=w678:u32)
                        n353 = Subtract(x=w675, y=w664) -> (x-y=w674:u32)
                        n354 = Subtract(x=w678, y=w663) -> (x-y=w677:u32)
                        n355 = Increment(x=w674) -> (x+1=w671:u32)
                      }
                      frame 5 {
                        n356 = Add(x=w685, y=w684) -> (x+y=w683:u32)
                        n357 = Add(x=w682, y=w681) -> (x+y=w680:u32)
                        n358 = Add(x=w687, y=w680) -> (x+y=w688:u32)
                        n359 = Subtract(x=w688, y=w679) -> (x-y=w686:u32)
                      }
                      frame 6 {
                        n360 = Add(x=w690, y=w689) -> (x+y=w691:u32)
                        n361 = Quotient & Remainder(x=w696, y=u32 2) -> (floor(x/y)=w698:u32)  [unwired: 1 out]
                        n362 = Add(x=w698, y=w691) -> (x+y=w701:u32)
                        n363 = Add(x=w694, y=w692) -> (x+y=w695:u32)
                        n364 = Add(x=w703, y=w695) -> (x+y=w704:u32)
                        n365 = Subtract(x=w701, y=w692) -> (x-y=w700:u32)
                        n366 = Subtract(x=w704, y=w693) -> (x-y=w702:u32)
                        n367 = Increment(x=w700) -> (x+1=w697:u32)
                      }
                      frame 7 {
                        n368 = Add(x=w710, y=w705) -> (x+y=w709:u32)
                        n369 = Add(x=w708, y=w705) -> (x+y=w706:u32)
                        n370 = Add(x=w711, y=w709) -> (x+y=w713:u32)
                        n371 = Add(x=w715, y=w706) -> (x+y=w716:u32)
                        n372 = Subtract(x=w713, y=w707) -> (x-y=w712:u32)
                        n373 = Subtract(x=w716, y=w707) -> (x-y=w714:u32)
                      }
                    }
                    n374 = property class="Bool"(reference=w622, "Left"=w620, "Top"=w618) -> ()  [unwired: 1 in, 2 out]
                  }
                }
              }
            }
            frame Error {
              n375 = To More Specific Class(target class=w791, reference=w793) -> (specific class reference=w795:refnum<vi>, error out=w794:errorcluster)  [unwired: 1 in]
              n376 = case shown="No Error" w794 {
                tunnel: w795 -> [w805 _]
                tunnel: w792 -> [w804 _]
                tunnel: w790 -> [w803 _]
                tunnel: w789 -> [w802 _]
                tunnel: w788 -> [w801 _]
                tunnel: w787 -> [w800 _]
                tunnel: w786 -> [w799 _]
                tunnel: w785 -> [w798 _]
                tunnel: w784 -> [w797 _]
                tunnel: w783 -> [w796 _]
                frame No Error {
                  n377 = Unbundle(w799) -> ("Width"=w807:u32, "Height"=w806:u32)
                  n378 = case shown="True" w798 {
                    tunnel: w801 -> [w821 w1012]
                    tunnel: w805 -> [_ w1011]
                    tunnel: w803 -> [w856 w987]
                    tunnel: w800 -> [_ w1009]
                    tunnel: w807 -> [_ w1008]
                    tunnel: w806 -> [_ w1007]
                    tunnel: w797 -> [_ w1006]
                    tunnel: w796 -> [_ w1005]
                    tunnel: w804 -> [w850 w992]
                    tunnel: w802 -> [_ w981]
                    frame False {
                      w811 = u32 20 ("y")
                      w816 = u32 10 ("y")
                      w835 = u32 32 ("y")
                      # "right\nbottom"
                      # "left\ntop"
                      # "right\nbottom"
                      # "left\ntop"
                      n379 = property class="Clust"(reference=w850) -> ("Height"=w812:u32, "Width"=w813:u32, "Left"=w820:i32, "Top"=w818:i32)  [unwired: 1 in, 2 out]
                      n380 = Add(x=w820, y=w813) -> (x+y=w837:u32)
                      n381 = Add(x=w818, y=w812) -> (x+y=w836:u32)
                      n382 = Add(x=w820, y=w816) -> (x+y=w819:u32)
                      n383 = Add(x=w818, y=w816) -> (x+y=w817:u32)
                      n384 = Decrement(x=w812) -> (x-1=w849:u32)
                      n385 = Bundle(w837, w836) -> (w855:cluster{u32, u32})  [unwired: 1 in]
                      n386 = Bundle("Left"=w820, "Top"=w818) -> (w854:cluster{"Left":i32, "Top":i32})  [unwired: 1 in]
                      n387 = Decrement(x=w813) -> (x-1=w845:u32)
                      n388 = Subtract(x=w813, y=w811) -> (x-y=w815:u32)
                      n389 = Subtract(x=w812, y=w811) -> (x-y=w814:u32)
                      n390 = Decrement(x=w849) -> (x-1=w848:u32)
                      n391 = Decrement(x=w845) -> (x-1=w844:u32)
                      n392 = Add(x=w819, y=w815) -> (x+y=w827:u32)
                      n393 = Decrement(x=w848) -> (x-1=w847:u32)
                      n394 = Add(x=w817, y=w814) -> (x+y=w828:u32)
                      n395 = Decrement(x=w844) -> (x-1=w843:u32)
                      n396 = Decrement(x=w847) -> (x-1=w846:u32)
                      n397 = Less?(x=w812, y=w835) -> (x < y?=w834:bool)
                      n398 = Less?(x=w813, y=w835) -> (x < y?=w833:bool)
                      n399 = Bundle(w827, w828) -> (w822:cluster{u32, u32})  [unwired: 1 in]
                      n400 = Bundle(w819, w817) -> (w823:cluster{u32, u32})  [unwired: 1 in]
                      n401 = Decrement(x=w843) -> (x-1=w842:u32)
                      n402 = Decrement(x=w846) -> (x-1=w841:u32)
                      n403 = Or(x=w834, y=w833) -> (x .or. y?=w832:bool)
                      n404 = Decrement(x=w842) -> (x-1=w839:u32)
                      n405 = Decrement(x=w841) -> (x-1=w840:u32)
                      n406 = In Range and Coerce(upper limit=w855, x=w821, lower limit=w854) -> (In Range?=w853:cluster{"Horizontal":bool, "Vertical":bool})  [unwired: 1 out]
                      n407 = In Range and Coerce(upper limit=w822, x=w821, lower limit=w823) -> (In Range?=w824:cluster{"Horizontal":bool, "Vertical":bool})  [unwired: 1 out]
                      n408 = Decrement(x=w839) -> (x-1=w838:u32)
                      n409 = Unbundle(w853) -> ("Horizontal"=w852:bool, "Vertical"=w851:bool)
                      n410 = Unbundle(w824) -> ("Horizontal"=w825:bool, "Vertical"=w826:bool)
                      n411 = And(x=w852, y=w851) -> (x .and. y?=w809:bool)
                      n412 = And(x=w825, y=w826) -> (x .and. y?=w808:bool)
                      n413 = Exclusive Or(1:w808, 2:w809) -> (0:w810:bool)
                      n414 = case shown="False" w832 {
                        tunnel: [u32 1 ("y") u32 2 ("y")] -> w831
                        tunnel: [u32 4 ("y") u32 8 ("y")] -> w829
                        tunnel: [u32 2 ("y") u32 4 ("y")] -> w830
                        frame True {
                        }
                        frame False {
                        }
                      }
                      n415 = case shown="True" w810 {
                        tunnel: w856 -> [w863 w873]
                        tunnel: w840 -> [_ w872]
                        tunnel: w838 -> [_ w871]
                        tunnel: w820 -> [_ w870]
                        tunnel: w818 -> [_ w869]
                        tunnel: w831 -> [_ w868]
                        tunnel: w830 -> [_ w867]
                        tunnel: w829 -> [_ w866]
                        frame False {
                          n416 = for {
                            tunnel: w863 -> [w865] mode=indexing
                            n417 = property class="Bool"(reference=w865, "Visible"=FALSE) -> ()  [unwired: 1 in, 2 out]
                          }
                        }
                        frame True {
                          n418 = for {
                            tunnel: w873 -> [w886] mode=indexing
                            tunnel: w870 -> [w883]
                            tunnel: w869 -> [w882]
                            tunnel: w872 -> [w881]
                            tunnel: w871 -> [w880]
                            tunnel: w868 -> [w878]
                            tunnel: w866 -> [w877]
                            tunnel: w867 -> [w876]
                            tunnel: w866 -> [w875]
                            i -> [w885]
                            n419 = case shown="2" w885 {
                              tunnel: [w892 w899 w911 w917 w941 w947 w961 w976] -> w884
                              tunnel: w883 -> [w888 w898 w907 w919 w930 w949 w954 w974]
                              tunnel: [w891 w895 w914 w922 w935 w950 w966 w978] -> w874
                              tunnel: w882 -> [w887 w897 w909 w918 w932 w946 w958 w972]
                              tunnel: w881 -> [_ _ _ w921 w934 w951 w967 w979]
                              tunnel: w880 -> [_ w902 w912 _ w940 _ w960 w975]
                              tunnel: w878 -> [w890 w894 w906 w916 w931 w948 w953 _]
                              tunnel: w876 -> [w889 w893 w905 w915 w928 w945 w956 w969]
                              tunnel: w875 -> [_ _ w910 _ w927 w943 w957 w971]
                              frame 0, Default {
                                n420 = Add(x=w888, y=w890) -> (x+y=w892:u32)
                                n421 = Add(x=w887, y=w889) -> (x+y=w891:u32)
                              }
                              frame 1 {
                                n422 = Quotient & Remainder(x=w902, y=u32 2) -> (floor(x/y)=w900:u32)  [unwired: 1 out]
                                n423 = Add(x=w898, y=w894) -> (x+y=w896:u32)
                                n424 = Add(x=w900, y=w896) -> (x+y=w904:u32)
                                n425 = Subtract(x=w904, y=w893) -> (x-y=w903:u32)
                                n426 = Add(x=w897, y=w893) -> (x+y=w895:u32)
                                n427 = Increment(x=w903) -> (x+1=w899:u32)
                              }
                              frame 2 {
                                n428 = Add(x=w907, y=w906) -> (x+y=w908:u32)
                                n429 = Add(x=w912, y=w908) -> (x+y=w913:u32)
                                n430 = Subtract(x=w913, y=w910) -> (x-y=w911:u32)
                                n431 = Add(x=w909, y=w905) -> (x+y=w914:u32)
                              }
                              frame 3 {
                                n432 = Quotient & Remainder(x=w921, y=u32 2) -> (floor(x/y)=w923:u32)  [unwired: 1 out]
                                n433 = Add(x=w918, y=w916) -> (x+y=w920:u32)
                                n434 = Add(x=w919, y=w916) -> (x+y=w917:u32)
                                n435 = Add(x=w923, y=w920) -> (x+y=w926:u32)
                                n436 = Subtract(x=w926, y=w915) -> (x-y=w925:u32)
                                n437 = Increment(x=w925) -> (x+1=w922:u32)
                              }
                              frame 4 {
                                n438 = Quotient & Remainder(x=w934, y=u32 2) -> (floor(x/y)=w936:u32)  [unwired: 1 out]
                                n439 = Add(x=w932, y=w931) -> (x+y=w933:u32)
                                n440 = Add(x=w936, y=w933) -> (x+y=w939:u32)
                                n441 = Add(x=w930, y=w928) -> (x+y=w929:u32)
                                n442 = Add(x=w940, y=w929) -> (x+y=w942:u32)
                                n443 = Subtract(x=w939, y=w928) -> (x-y=w938:u32)
                                n444 = Subtract(x=w942, y=w927) -> (x-y=w941:u32)
                                n445 = Increment(x=w938) -> (x+1=w935:u32)
                              }
                              frame 5 {
                                n446 = Add(x=w949, y=w948) -> (x+y=w947:u32)
                                n447 = Add(x=w946, y=w945) -> (x+y=w944:u32)
                                n448 = Add(x=w951, y=w944) -> (x+y=w952:u32)
                                n449 = Subtract(x=w952, y=w943) -> (x-y=w950:u32)
                              }
                              frame 6 {
                                n450 = Add(x=w954, y=w953) -> (x+y=w955:u32)
                                n451 = Quotient & Remainder(x=w960, y=u32 2) -> (floor(x/y)=w962:u32)  [unwired: 1 out]
                                n452 = Add(x=w962, y=w955) -> (x+y=w965:u32)
                                n453 = Add(x=w958, y=w956) -> (x+y=w959:u32)
                                n454 = Add(x=w967, y=w959) -> (x+y=w968:u32)
                                n455 = Subtract(x=w965, y=w956) -> (x-y=w964:u32)
                                n456 = Subtract(x=w968, y=w957) -> (x-y=w966:u32)
                                n457 = Increment(x=w964) -> (x+1=w961:u32)
                              }
                              frame 7 {
                                n458 = Add(x=w974, y=w969) -> (x+y=w973:u32)
                                n459 = Add(x=w972, y=w969) -> (x+y=w970:u32)
                                n460 = Add(x=w975, y=w973) -> (x+y=w977:u32)
                                n461 = Add(x=w979, y=w970) -> (x+y=w980:u32)
                                n462 = Subtract(x=w977, y=w971) -> (x-y=w976:u32)
                                n463 = Subtract(x=w980, y=w971) -> (x-y=w978:u32)
                              }
                            }
                            n464 = property class="Bool"(reference=w886, "Visible"=TRUE, "Left"=w884, "Top"=w874, "Height"=w877, "Width"=w877) -> ()  [unwired: 1 in, 2 out]
                          }
                        }
                      }
                    }
                    frame True {
                      w984 = u32 2 ("y")
                      n465 = Subtract(x=w1012, y=w981) -> (x-y=w1010:T3)
                      n466 = case shown="\"size 7\"" w1009 {
                        tunnel: w1011 -> [_ w1125 w1135 w1151]
                        tunnel: w1010 -> [_ w1127 w1137 w1152]
                        tunnel: w1008 -> [_ w1124 _ w1147]
                        tunnel: w1007 -> [_ _ w1134 w1150]
                        tunnel: w1006 -> [_ w1123 w1132 w1144]
                        tunnel: w1005 -> [_ w1122 w1131 w1143]
                        frame "False", Default {
                        }
                        frame "size 2", "size 4" {
                          n467 = Unbundle(w1127) -> ("Horizontal"=w1119:i32)  [unwired: 1 out]
                          n468 = Unbundle(w1122) -> ("Right"=w1120:i16)  [unwired: 3 out]
                          n469 = Add(x=w1124, y=w1119) -> (x+y=w1126:u32)
                          n470 = Add(x=w1120, y=w1119) -> (x+y=w1118:i32)
                          n471 = property class="Bool"(reference=w1125, "Width"=w1126) -> ()  [unwired: 1 in, 2 out]
                          n472 = Bundle(cluster=w1122, "Right"=w1118) -> (w1121:T1)  [unwired: 3 in]
                          n473 = property class="VI"(reference=w1123, "Front Panel.WinBounds"=w1121) -> ()  [unwired: 1 in, 2 out]
                        }
                        frame "size 6" {
                          n474 = Unbundle(w1137) -> ("Vertical"=w1130:i32)  [unwired: 1 out]
                          n475 = Unbundle(w1131) -> ("Bottom"=w1129:i16)  [unwired: 3 out]
                          n476 = Add(x=w1134, y=w1130) -> (x+y=w1136:u32)
                          n477 = property class="Bool"(reference=w1135, "Height"=w1136) -> ()  [unwired: 1 in, 2 out]
                          n478 = Add(x=w1129, y=w1130) -> (x+y=w1128:i32)
                          n479 = Bundle(cluster=w1131, "Bottom"=w1128) -> (w1133:T1)  [unwired: 3 in]
                          n480 = property class="VI"(reference=w1132, "Front Panel.WinBounds"=w1133) -> ()  [unwired: 1 in, 2 out]
                        }
                        frame "size 7" {
                          n481 = Unbundle(w1143) -> ("Right"=w1145:i16, "Bottom"=w1140:i16)  [unwired: 2 out]
                          n482 = Unbundle(w1152) -> ("Horizontal"=w1139:i32, "Vertical"=w1138:i32)
                          n483 = Add(x=w1139, y=w1147) -> (x+y=w1148:u32)
                          n484 = Add(x=w1150, y=w1138) -> (x+y=w1149:u32)
                          n485 = property class="Bool"(reference=w1151, "Width"=w1148, "Height"=w1149) -> ()  [unwired: 1 in, 2 out]
                          n486 = Add(x=w1145, y=w1139) -> (x+y=w1142:i32)
                          n487 = Add(x=w1140, y=w1138) -> (x+y=w1141:i32)
                          n488 = Bundle(cluster=w1143, "Right"=w1142, "Bottom"=w1141) -> (w1146:T1)  [unwired: 2 in]
                          n489 = property class="VI"(reference=w1144, "Front Panel.WinBounds"=w1146) -> ()  [unwired: 1 in, 2 out]
                        }
                      }
                      n490 = property class="Clust"(reference=w992) -> ("Height"=w1004:u32, "Width"=w1003:u32, "Left"=w989:i32, "Top"=w988:i32)  [unwired: 1 in, 2 out]
                      n491 = Decrement(x=w1004) -> (x-1=w1002:u32)
                      n492 = Decrement(x=w1003) -> (x-1=w998:u32)
                      n493 = Decrement(x=w1002) -> (x-1=w1001:u32)
                      n494 = Decrement(x=w998) -> (x-1=w997:u32)
                      n495 = Decrement(x=w1001) -> (x-1=w1000:u32)
                      n496 = Decrement(x=w997) -> (x-1=w996:u32)
                      n497 = Decrement(x=w1000) -> (x-1=w999:u32)
                      n498 = Decrement(x=w996) -> (x-1=w995:u32)
                      n499 = Decrement(x=w999) -> (x-1=w994:u32)
                      n500 = Decrement(x=w995) -> (x-1=w993:u32)
                      n501 = Decrement(x=w994) -> (x-1=w991:u32)
                      n502 = Decrement(x=w993) -> (x-1=w990:u32)
                      n503 = Index Array(array=w987) -> (element=w986:refnum<vi>)  [unwired: 1 in]
                      n504 = property class="Bool"(reference=w986) -> ("Height"=w985:u32)  [unwired: 1 in, 2 out]
                      n505 = Quotient & Remainder(x=w985, y=w984) -> (floor(x/y)=w983:u32)  [unwired: 1 out]
                      n506 = Quotient & Remainder(x=w983, y=w984) -> (floor(x/y)=w982:u32)  [unwired: 1 out]
                      n507 = for {
                        tunnel: w987 -> [w1023] mode=indexing
                        tunnel: w989 -> [w1020]
                        tunnel: w988 -> [w1019]
                        tunnel: w991 -> [w1018]
                        tunnel: w990 -> [w1017]
                        tunnel: w982 -> [w1016]
                        tunnel: w983 -> [w1015]
                        tunnel: w985 -> [w1014]
                        i -> [w1022]
                        n508 = case shown="5" w1022 {
                          tunnel: [w1029 w1036 w1048 w1054 w1078 w1084 w1098 w1113] -> w1021
                          tunnel: w1020 -> [w1025 w1035 w1044 w1056 w1067 w1086 w1091 w1111]
                          tunnel: [w1028 w1032 w1051 w1059 w1072 w1087 w1103 w1115] -> w1013
                          tunnel: w1019 -> [w1024 w1034 w1046 w1055 w1069 w1083 w1095 w1109]
                          tunnel: w1018 -> [_ _ _ w1058 w1071 w1088 w1104 w1116]
                          tunnel: w1017 -> [_ w1039 w1049 _ w1077 _ w1097 w1112]
                          tunnel: w1016 -> [w1027 w1031 w1043 w1053 w1068 w1085 w1090 _]
                          tunnel: w1015 -> [w1026 w1030 w1042 w1052 w1065 w1082 w1093 w1106]
                          tunnel: w1014 -> [_ _ w1047 _ w1064 w1080 w1094 w1108]
                          frame 0, Default {
                            n509 = Add(x=w1025, y=w1027) -> (x+y=w1029:u32)
                            n510 = Add(x=w1024, y=w1026) -> (x+y=w1028:u32)
                          }
                          frame 1 {
                            n511 = Quotient & Remainder(x=w1039, y=u32 2) -> (floor(x/y)=w1037:u32)  [unwired: 1 out]
                            n512 = Add(x=w1035, y=w1031) -> (x+y=w1033:u32)
                            n513 = Add(x=w1037, y=w1033) -> (x+y=w1041:u32)
                            n514 = Add(x=w1034, y=w1030) -> (x+y=w1032:u32)
                            n515 = Subtract(x=w1041, y=w1030) -> (x-y=w1040:u32)
                            n516 = Increment(x=w1040) -> (x+1=w1036:u32)
                          }
                          frame 2 {
                            n517 = Add(x=w1044, y=w1043) -> (x+y=w1045:u32)
                            n518 = Add(x=w1049, y=w1045) -> (x+y=w1050:u32)
                            n519 = Add(x=w1046, y=w1042) -> (x+y=w1051:u32)
                            n520 = Subtract(x=w1050, y=w1047) -> (x-y=w1048:u32)
                          }
                          frame 3 {
                            n521 = Quotient & Remainder(x=w1058, y=u32 2) -> (floor(x/y)=w1060:u32)  [unwired: 1 out]
                            n522 = Add(x=w1055, y=w1053) -> (x+y=w1057:u32)
                            n523 = Add(x=w1056, y=w1053) -> (x+y=w1054:u32)
                            n524 = Add(x=w1060, y=w1057) -> (x+y=w1063:u32)
                            n525 = Subtract(x=w1063, y=w1052) -> (x-y=w1062:u32)
                            n526 = Increment(x=w1062) -> (x+1=w1059:u32)
                          }
                          frame 4 {
                            n527 = Quotient & Remainder(x=w1071, y=u32 2) -> (floor(x/y)=w1073:u32)  [unwired: 1 out]
                            n528 = Add(x=w1069, y=w1068) -> (x+y=w1070:u32)
                            n529 = Add(x=w1073, y=w1070) -> (x+y=w1076:u32)
                            n530 = Add(x=w1067, y=w1065) -> (x+y=w1066:u32)
                            n531 = Add(x=w1077, y=w1066) -> (x+y=w1079:u32)
                            n532 = Subtract(x=w1076, y=w1065) -> (x-y=w1075:u32)
                            n533 = Subtract(x=w1079, y=w1064) -> (x-y=w1078:u32)
                            n534 = Increment(x=w1075) -> (x+1=w1072:u32)
                          }
                          frame 5 {
                            n535 = Add(x=w1086, y=w1085) -> (x+y=w1084:u32)
                            n536 = Add(x=w1083, y=w1082) -> (x+y=w1081:u32)
                            n537 = Add(x=w1088, y=w1081) -> (x+y=w1089:u32)
                            n538 = Subtract(x=w1089, y=w1080) -> (x-y=w1087:u32)
                          }
                          frame 6 {
                            n539 = Add(x=w1091, y=w1090) -> (x+y=w1092:u32)
                            n540 = Quotient & Remainder(x=w1097, y=u32 2) -> (floor(x/y)=w1099:u32)  [unwired: 1 out]
                            n541 = Add(x=w1099, y=w1092) -> (x+y=w1102:u32)
                            n542 = Add(x=w1095, y=w1093) -> (x+y=w1096:u32)
                            n543 = Add(x=w1104, y=w1096) -> (x+y=w1105:u32)
                            n544 = Subtract(x=w1102, y=w1093) -> (x-y=w1101:u32)
                            n545 = Subtract(x=w1105, y=w1094) -> (x-y=w1103:u32)
                            n546 = Increment(x=w1101) -> (x+1=w1098:u32)
                          }
                          frame 7 {
                            n547 = Add(x=w1111, y=w1106) -> (x+y=w1110:u32)
                            n548 = Add(x=w1109, y=w1106) -> (x+y=w1107:u32)
                            n549 = Add(x=w1112, y=w1110) -> (x+y=w1114:u32)
                            n550 = Add(x=w1116, y=w1107) -> (x+y=w1117:u32)
                            n551 = Subtract(x=w1114, y=w1108) -> (x-y=w1113:u32)
                            n552 = Subtract(x=w1117, y=w1108) -> (x-y=w1115:u32)
                          }
                        }
                        n553 = property class="Bool"(reference=w1023, "Left"=w1021, "Top"=w1013) -> ()  [unwired: 1 in, 2 out]
                      }
                    }
                  }
                }
                frame Error {
                }
              }
            }
          }
        }
      }
    }
    frame True {
    }
  }
